vi "FTW-File-FileInfo.vi"(0 "Filepath":path, 11 "error in":errorcluster) -> (6 "Filesize (MB)":string, 15 "error out":errorcluster)   [LabVIEW 2015]
uses:
  string/FTW-STR-DisplayFormat-Bytes.ctl
panel:
  # "Inputs"
  # "Outputs"
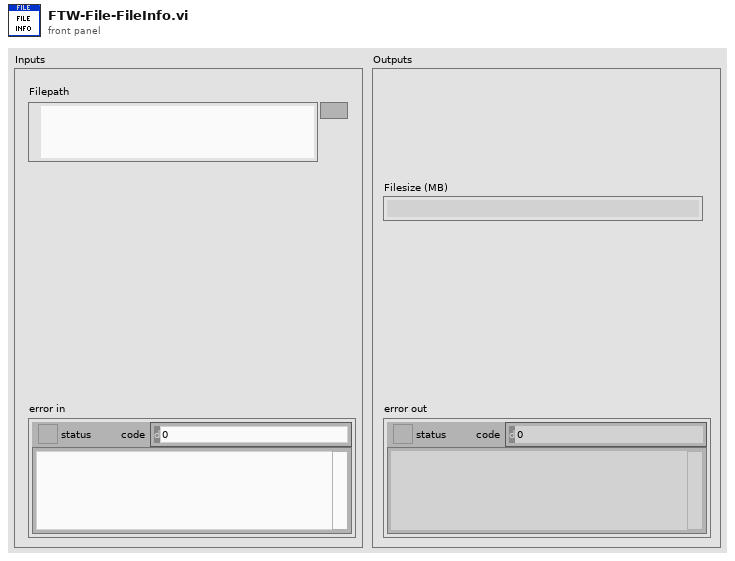
[diagram p1: front panel]
types:
  T1 = typedef "FTW-STR-DisplayFormat-Bytes.ctl" = enum16{"Auto", "Plain Bytes", "000 bytes", "0.00kB", "0.00MB", "0.00GB", "0.00TB", "Transfer Rate"}
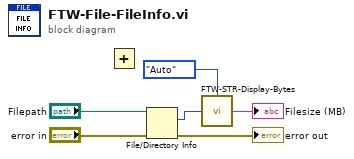
[diagram p0: block diagram]
diagram:
  n1 = Add() -> ()  [unwired: 2 in, 1 out]
  n2 = File/Directory Info(path="Filepath", error in="error in") -> (size=w3:i64, error out=→"error out":errorcluster)  [unwired: 5 out]
  n3 = call "FTW-STR-Display-Bytes.vi"("Bytes"=w3, "Display Format"=FTW-STR-DisplayFormat-Bytes."Auto") -> ("Display"=→"Filesize (MB)":string)
